vi "Test Get Active Plugins.vi"(8 "error in (no error)":errorcluster, 11 "Configuration Manager Test in":refnum<class "Configuration Manager Test.lvclass">) -> (0 "error out":errorcluster, 3 "Configuration Manager Test out":refnum<class "Configuration Manager Test.lvclass">)   [LabVIEW 2020, in "Configuration Manager Test.lvclass"]
uses:
  Configuration Manager Test.lvclass
  C:/Program Files (x86)/National Instruments/LabVIEW 2020/vi.lib/Astemes/LUnit/Test Case.lvclass
  <vilib>/Astemes/LUnit/Test Case.lvclass/Test Case.ctl
  b78b68b9-28ec-4fcb-9b61-f705c7f0904e.vi
  <vilib>/Astemes/LUnit/Palette/Pass.vi
  <vilib>/Astemes/LUnit/Palette/Fail.vi
  <vilib>/Astemes/LUnit/Compare Variants.vi
  <vilib>/Astemes/LUnit/Describe Comparison.vi
  <vilib>/Astemes/LUnit/Set Assertion Type.vi
  <vilib>/Astemes/LUnit/Add test result.vi
  <vilib>/Astemes/LUnit/Variant to string.vi
  <vilib>/Astemes/LUnit/LUnit Record Assertion Result.vi
  <vilib>/Astemes/LUnit/LUnit Aggregate Assertion Results.vi
  <vilib>/Astemes/LUnit/Method Result/LUnit Merge Status.vi
  <vilib>/Astemes/LUnit/LUnit Concatenate result strings.vi
  <vilib>/Utility/Data Type/Get Type Information.vi
  <vilib>/Utility/LVClass/Get LV Class Name.vi
  Configuration Manager Test.lvclass/Configuration Manager Test.ctl
  source/User Interface/Configuration Manager/Configuration Manager.lvclass
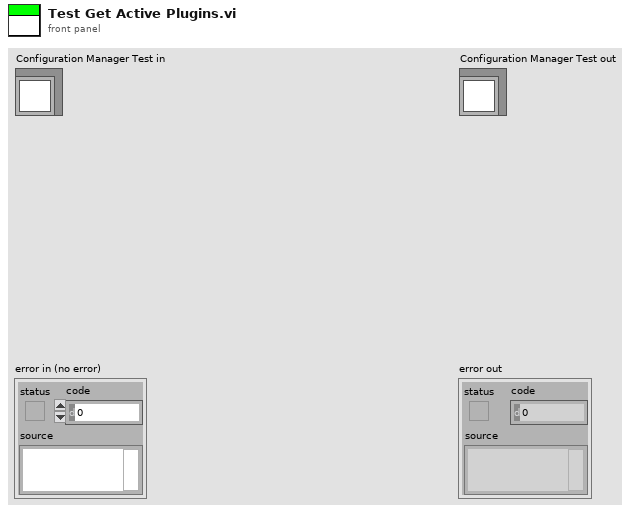
[diagram p1: front panel]
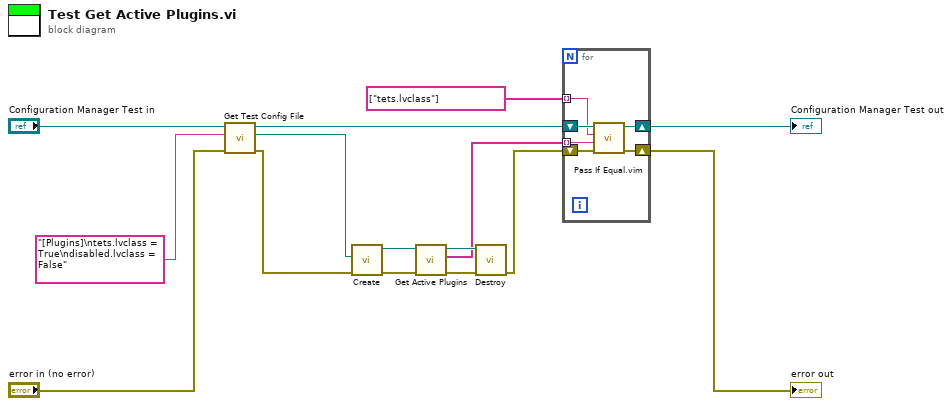
[diagram p0: block diagram]
diagram:
  n1 = call "Get Test Config File.vi"("error in (no error)"="error in (no error)", "File Content"="[Plugins]\ntets.lvclass = True\ndisabled.lvclass = False", "Configuration Manager Test in"="Configuration Manager Test in") -> ("error out"=w8:errorcluster, "File Path"=w3:path, "Configuration Manager Test out"=w5:refnum<class "Configuration Manager Test.lvclass">)  [unwired: 6 in]
  n2 = call "Create.vi"("error in (no error)"=w8, "configuration file path"=w3) -> ("error out"=w11:errorcluster, "Configuration Manager out"=w12:refnum<class "Configuration Manager.lvclass">)  [unwired: 8 in]
  n3 = call "Get Active Plugins.vi"("error in (no error)"=w11, "Configuration Manager In"=w12) -> ("error out"=w9:errorcluster, "Plugins"=w2:string[], "Configuration Manager Out"=w10:refnum<class "Configuration Manager.lvclass">)  [unwired: 7 in]
  n4 = call "Destroy.vi"("error in (no error)"=w9, "Configuration Manager In"=w10) -> ("error out"=w7:errorcluster)  [unwired: 9 in]
  n5 = for {
    tunnel: w2 -> [w17] mode=indexing
    tunnel: string[] ["tets.lvclass"] -> [w16] mode=indexing
    shift-right: [w20] -> w6
    shift-left: w7 -> [w21]
    shift-right: [w18] -> w4
    shift-left: w5 -> [w19]
    n6 = call "Pass If Equal.vim"("error in (no error)"=w21, "Actual"=w17, "Expected"=w16, "LUnit Test Case In"=w19) -> ("error out"=w20:errorcluster, "LUnit Test Case Out"=w18:refnum<class "Configuration Manager Test.lvclass">)  [unwired: 6 in]
  }
  "error out" <- w6
  "Configuration Manager Test out" <- w4
